vi "real pool auto routine.vi"(0 "ROI Descriptor (Geometric Matching 1)":T4={"Global Rectangle"=[20, 20, 1364, 1012], "Contours"=[{"ID"=enum."External", "Type"=3, "Coordinates"=[20, 20, 1364, 1012]}]} {"Contours"."Type" items=["No Selection", "Point", "Line", "Rectangle", "Oval", "Polygon", "Freehand Region", "Annulus", "Unused2", "Unused3", "Broken Line", "Freehand Line", "Rotated Rectangle"]}, 1 "Settings (Geometric Matching 1)":T3={"Curve Parameters"={"Extraction Mode"=0, "Edge Threshold"=75, "Edge Filter Size"=1, "Min Length"=25, "Row Search Step Size"=15, "Col Search Step Size"=15, "Max Endpoint Gap"=10, "Closed"=FALSE, "Subpixel"=FALSE}, "Match Mode"={"Rotation"=TRUE, "Scale"=FALSE, "Occlusion"=TRUE, "Reserved"=FALSE, "Reserved"=FALSE, "Reserved"=FALSE}, "Range Settings"=[{"Match Constraints"=0, "Min"=0.0, "Max"=360.0}, {"Match Constraints"=2, "Min"=0.0, "Max"=25.0}], "Number of Matches"=1, "Minimum Match Score"=800.0, "SubPixel Accuracy"=FALSE, "Adv. Geometric Match Options 2"=[{"Setup Data Item"=21, "Item Value"=0.0}, {"Setup Data Item"=22, "Item Value"=1.0}]} {"Curve Parameters"."Extraction Mode" items=["Normal", "Uniform Regions"]; "Curve Parameters"."Edge Filter Size" items=["Fine", "Normal", "Contour Tracing"]; "Curve Parameters"."Max Endpoint Gap" min=0; "Curve Parameters"."Col Search Step Size" min=1 max=255 step=1; "Curve Parameters"."Row Search Step Size" min=1 max=255 step=1; "Curve Parameters"."Min Length" min=0; "Curve Parameters"."Edge Threshold" min=1 max=350 step=1; "Range Settings"."Max" format="%.2f"; "Range Settings"."Min" format="%.2f"; "Range Settings"."Match Constraints" items=["Rotation Angle (degrees)", "Scale Factor (%)", "Occlusion (%)"]; "Adv. Geometric Match Options 2"."Setup Data Item" items=["Curve Extraction Mode", "Curve Edge Threshold", "Curve Edge Filter Size", "Min Curve Length", "Curve Row Search Step Size", "Curve Col Search Step Size", "Curve Max Endpoint Gap", "Extract Closed Curves", "Enable Subpixel Curve Extraction", "Enable Correlation Score", "Enable Subpixel Accuracy", "Subpixel Iterations", "Subpixel Tolerance", "Initial Match List Length", "Enable Target Template Curve Score", "Min Match Separation Distance", "Min Match Separation Angle", "Min Match Separation Scale", "Max Match Overlap", "Enable Coarse Result", "Enable Calibration Support", "Enable Contrast Reversal", "Search Strategy", "Refinement Match Factor", "Subpixel Match Factor"]}, 2 "Template File Path (Geometric Matching 1)":path=path "C:/Users/GARLAND/Documents/Projects/Robotics I/Robotics I 3390 2012/Final project/Labview/Real Pool navigation/real pool location templete.png", 3 "ROI Descriptor (Geometric Matching 2)":T4={"Global Rectangle"=[20, 20, 1364, 1012], "Contours"=[{"ID"=enum."External", "Type"=3, "Coordinates"=[20, 20, 1364, 1012]}]} {"Contours"."Type" items=["No Selection", "Point", "Line", "Rectangle", "Oval", "Polygon", "Freehand Region", "Annulus", "Unused2", "Unused3", "Broken Line", "Freehand Line", "Rotated Rectangle"]}, 4 "Settings (Geometric Matching 2)":T3={"Curve Parameters"={"Extraction Mode"=0, "Edge Threshold"=75, "Edge Filter Size"=1, "Min Length"=25, "Row Search Step Size"=15, "Col Search Step Size"=15, "Max Endpoint Gap"=10, "Closed"=FALSE, "Subpixel"=FALSE}, "Match Mode"={"Rotation"=TRUE, "Scale"=FALSE, "Occlusion"=TRUE, "Reserved"=FALSE, "Reserved"=FALSE, "Reserved"=FALSE}, "Range Settings"=[{"Match Constraints"=0, "Min"=0.0, "Max"=360.0}, {"Match Constraints"=2, "Min"=0.0, "Max"=25.0}], "Number of Matches"=1, "Minimum Match Score"=800.0, "SubPixel Accuracy"=FALSE, "Adv. Geometric Match Options 2"=[{"Setup Data Item"=21, "Item Value"=0.0}, {"Setup Data Item"=22, "Item Value"=1.0}]} {"Curve Parameters"."Extraction Mode" items=["Normal", "Uniform Regions"]; "Curve Parameters"."Edge Filter Size" items=["Fine", "Normal", "Contour Tracing"]; "Curve Parameters"."Max Endpoint Gap" min=0; "Curve Parameters"."Col Search Step Size" min=1 max=255 step=1; "Curve Parameters"."Row Search Step Size" min=1 max=255 step=1; "Curve Parameters"."Min Length" min=0; "Curve Parameters"."Edge Threshold" min=1 max=350 step=1; "Range Settings"."Max" format="%.2f"; "Range Settings"."Min" format="%.2f"; "Range Settings"."Match Constraints" items=["Rotation Angle (degrees)", "Scale Factor (%)", "Occlusion (%)"]; "Adv. Geometric Match Options 2"."Setup Data Item" items=["Curve Extraction Mode", "Curve Edge Threshold", "Curve Edge Filter Size", "Min Curve Length", "Curve Row Search Step Size", "Curve Col Search Step Size", "Curve Max Endpoint Gap", "Extract Closed Curves", "Enable Subpixel Curve Extraction", "Enable Correlation Score", "Enable Subpixel Accuracy", "Subpixel Iterations", "Subpixel Tolerance", "Initial Match List Length", "Enable Target Template Curve Score", "Min Match Separation Distance", "Min Match Separation Angle", "Min Match Separation Scale", "Max Match Overlap", "Enable Coarse Result", "Enable Calibration Support", "Enable Contrast Reversal", "Search Strategy", "Refinement Match Factor", "Subpixel Match Factor"]}, 5 "Template File Path (Geometric Matching 2)":path=path "C:/Users/GARLAND/Documents/Projects/Robotics I/Robotics I 3390 2012/Final project/Labview/Real Pool navigation/real pool boat templete.png", 6 "ROI Descriptor (Geometric Matching 3)":T4={"Global Rectangle"=[20, 20, 1364, 1012], "Contours"=[{"ID"=enum."External", "Type"=3, "Coordinates"=[20, 20, 1364, 1012]}]} {"Contours"."Type" items=["No Selection", "Point", "Line", "Rectangle", "Oval", "Polygon", "Freehand Region", "Annulus", "Unused2", "Unused3", "Broken Line", "Freehand Line", "Rotated Rectangle"]}, 7 "error in":errorcluster, 8 "Settings (Geometric Matching 3)":T3={"Curve Parameters"={"Extraction Mode"=0, "Edge Threshold"=75, "Edge Filter Size"=1, "Min Length"=25, "Row Search Step Size"=15, "Col Search Step Size"=15, "Max Endpoint Gap"=10, "Closed"=FALSE, "Subpixel"=FALSE}, "Match Mode"={"Rotation"=TRUE, "Scale"=FALSE, "Occlusion"=TRUE, "Reserved"=FALSE, "Reserved"=FALSE, "Reserved"=FALSE}, "Range Settings"=[{"Match Constraints"=0, "Min"=0.0, "Max"=360.0}, {"Match Constraints"=2, "Min"=0.0, "Max"=25.0}], "Number of Matches"=1, "Minimum Match Score"=800.0, "SubPixel Accuracy"=FALSE, "Adv. Geometric Match Options 2"=[{"Setup Data Item"=21, "Item Value"=0.0}, {"Setup Data Item"=22, "Item Value"=1.0}]} {"Curve Parameters"."Extraction Mode" items=["Normal", "Uniform Regions"]; "Curve Parameters"."Edge Filter Size" items=["Fine", "Normal", "Contour Tracing"]; "Curve Parameters"."Max Endpoint Gap" min=0; "Curve Parameters"."Col Search Step Size" min=1 max=255 step=1; "Curve Parameters"."Row Search Step Size" min=1 max=255 step=1; "Curve Parameters"."Min Length" min=0; "Curve Parameters"."Edge Threshold" min=1 max=350 step=1; "Range Settings"."Max" format="%.2f"; "Range Settings"."Min" format="%.2f"; "Range Settings"."Match Constraints" items=["Rotation Angle (degrees)", "Scale Factor (%)", "Occlusion (%)"]; "Adv. Geometric Match Options 2"."Setup Data Item" items=["Curve Extraction Mode", "Curve Edge Threshold", "Curve Edge Filter Size", "Min Curve Length", "Curve Row Search Step Size", "Curve Col Search Step Size", "Curve Max Endpoint Gap", "Extract Closed Curves", "Enable Subpixel Curve Extraction", "Enable Correlation Score", "Enable Subpixel Accuracy", "Subpixel Iterations", "Subpixel Tolerance", "Initial Match List Length", "Enable Target Template Curve Score", "Min Match Separation Distance", "Min Match Separation Angle", "Min Match Separation Scale", "Max Match Overlap", "Enable Coarse Result", "Enable Calibration Support", "Enable Contrast Reversal", "Search Strategy", "Refinement Match Factor", "Subpixel Match Factor"]}, 9 "Template File Path (Geometric Matching 3)":path=path "C:/Users/GARLAND/Documents/Projects/Robotics I/Robotics I 3390 2012/Final project/Labview/Real Pool navigation/real pool bouy templete.png", 10 "ROI Descriptor (Geometric Matching 4)":T4={"Global Rectangle"=[20, 20, 1364, 1012], "Contours"=[{"ID"=enum."External", "Type"=3, "Coordinates"=[20, 20, 1364, 1012]}]} {"Contours"."Type" items=["No Selection", "Point", "Line", "Rectangle", "Oval", "Polygon", "Freehand Region", "Annulus", "Unused2", "Unused3", "Broken Line", "Freehand Line", "Rotated Rectangle"]}, 11 "Settings (Geometric Matching 4)":T3={"Curve Parameters"={"Extraction Mode"=0, "Edge Threshold"=75, "Edge Filter Size"=1, "Min Length"=25, "Row Search Step Size"=15, "Col Search Step Size"=15, "Max Endpoint Gap"=10, "Closed"=FALSE, "Subpixel"=FALSE}, "Match Mode"={"Rotation"=TRUE, "Scale"=FALSE, "Occlusion"=TRUE, "Reserved"=FALSE, "Reserved"=FALSE, "Reserved"=FALSE}, "Range Settings"=[{"Match Constraints"=0, "Min"=0.0, "Max"=360.0}, {"Match Constraints"=2, "Min"=0.0, "Max"=25.0}], "Number of Matches"=1, "Minimum Match Score"=800.0, "SubPixel Accuracy"=FALSE, "Adv. Geometric Match Options 2"=[{"Setup Data Item"=21, "Item Value"=0.0}, {"Setup Data Item"=22, "Item Value"=1.0}]} {"Curve Parameters"."Extraction Mode" items=["Normal", "Uniform Regions"]; "Curve Parameters"."Edge Filter Size" items=["Fine", "Normal", "Contour Tracing"]; "Curve Parameters"."Max Endpoint Gap" min=0; "Curve Parameters"."Col Search Step Size" min=1 max=255 step=1; "Curve Parameters"."Row Search Step Size" min=1 max=255 step=1; "Curve Parameters"."Min Length" min=0; "Curve Parameters"."Edge Threshold" min=1 max=350 step=1; "Range Settings"."Max" format="%.2f"; "Range Settings"."Min" format="%.2f"; "Range Settings"."Match Constraints" items=["Rotation Angle (degrees)", "Scale Factor (%)", "Occlusion (%)"]; "Adv. Geometric Match Options 2"."Setup Data Item" items=["Curve Extraction Mode", "Curve Edge Threshold", "Curve Edge Filter Size", "Min Curve Length", "Curve Row Search Step Size", "Curve Col Search Step Size", "Curve Max Endpoint Gap", "Extract Closed Curves", "Enable Subpixel Curve Extraction", "Enable Correlation Score", "Enable Subpixel Accuracy", "Subpixel Iterations", "Subpixel Tolerance", "Initial Match List Length", "Enable Target Template Curve Score", "Min Match Separation Distance", "Min Match Separation Angle", "Min Match Separation Scale", "Max Match Overlap", "Enable Coarse Result", "Enable Calibration Support", "Enable Contrast Reversal", "Search Strategy", "Refinement Match Factor", "Subpixel Match Factor"]}, 12 "Template File Path (Geometric Matching 4)":path=path "C:/Users/GARLAND/Documents/Projects/Robotics I/Robotics I 3390 2012/Final project/Labview/Real Pool navigation/real pool whale templete.png", 13 "ROI Descriptor (Geometric Matching 5)":T4={"Global Rectangle"=[20, 20, 1364, 1012], "Contours"=[{"ID"=enum."External", "Type"=3, "Coordinates"=[20, 20, 1364, 1012]}]} {"Contours"."Type" items=["No Selection", "Point", "Line", "Rectangle", "Oval", "Polygon", "Freehand Region", "Annulus", "Unused2", "Unused3", "Broken Line", "Freehand Line", "Rotated Rectangle"]}, 14 "Settings (Geometric Matching 5)":T3={"Curve Parameters"={"Extraction Mode"=0, "Edge Threshold"=75, "Edge Filter Size"=1, "Min Length"=25, "Row Search Step Size"=15, "Col Search Step Size"=15, "Max Endpoint Gap"=10, "Closed"=FALSE, "Subpixel"=FALSE}, "Match Mode"={"Rotation"=TRUE, "Scale"=FALSE, "Occlusion"=TRUE, "Reserved"=FALSE, "Reserved"=FALSE, "Reserved"=FALSE}, "Range Settings"=[{"Match Constraints"=0, "Min"=0.0, "Max"=360.0}, {"Match Constraints"=2, "Min"=0.0, "Max"=25.0}], "Number of Matches"=1, "Minimum Match Score"=800.0, "SubPixel Accuracy"=FALSE, "Adv. Geometric Match Options 2"=[{"Setup Data Item"=21, "Item Value"=0.0}, {"Setup Data Item"=22, "Item Value"=1.0}]} {"Curve Parameters"."Extraction Mode" items=["Normal", "Uniform Regions"]; "Curve Parameters"."Edge Filter Size" items=["Fine", "Normal", "Contour Tracing"]; "Curve Parameters"."Max Endpoint Gap" min=0; "Curve Parameters"."Col Search Step Size" min=1 max=255 step=1; "Curve Parameters"."Row Search Step Size" min=1 max=255 step=1; "Curve Parameters"."Min Length" min=0; "Curve Parameters"."Edge Threshold" min=1 max=350 step=1; "Range Settings"."Max" format="%.2f"; "Range Settings"."Min" format="%.2f"; "Range Settings"."Match Constraints" items=["Rotation Angle (degrees)", "Scale Factor (%)", "Occlusion (%)"]; "Adv. Geometric Match Options 2"."Setup Data Item" items=["Curve Extraction Mode", "Curve Edge Threshold", "Curve Edge Filter Size", "Min Curve Length", "Curve Row Search Step Size", "Curve Col Search Step Size", "Curve Max Endpoint Gap", "Extract Closed Curves", "Enable Subpixel Curve Extraction", "Enable Correlation Score", "Enable Subpixel Accuracy", "Subpixel Iterations", "Subpixel Tolerance", "Initial Match List Length", "Enable Target Template Curve Score", "Min Match Separation Distance", "Min Match Separation Angle", "Min Match Separation Scale", "Max Match Overlap", "Enable Coarse Result", "Enable Calibration Support", "Enable Contrast Reversal", "Search Strategy", "Refinement Match Factor", "Subpixel Match Factor"]}, 15 "Template File Path (Geometric Matching 5)":path=path "C:/Users/GARLAND/Documents/Projects/Robotics I/Robotics I 3390 2012/Final project/Labview/Real Pool navigation/real pool square templete.png", 16 "ROI Descriptor (Geometric Matching 6)":T4={"Global Rectangle"=[20, 20, 1364, 1012], "Contours"=[{"ID"=enum."External", "Type"=3, "Coordinates"=[20, 20, 1364, 1012]}]} {"Contours"."Type" items=["No Selection", "Point", "Line", "Rectangle", "Oval", "Polygon", "Freehand Region", "Annulus", "Unused2", "Unused3", "Broken Line", "Freehand Line", "Rotated Rectangle"]}, 17 "Settings (Geometric Matching 6)":T3={"Curve Parameters"={"Extraction Mode"=0, "Edge Threshold"=75, "Edge Filter Size"=1, "Min Length"=25, "Row Search Step Size"=15, "Col Search Step Size"=15, "Max Endpoint Gap"=10, "Closed"=FALSE, "Subpixel"=FALSE}, "Match Mode"={"Rotation"=TRUE, "Scale"=FALSE, "Occlusion"=TRUE, "Reserved"=FALSE, "Reserved"=FALSE, "Reserved"=FALSE}, "Range Settings"=[{"Match Constraints"=0, "Min"=0.0, "Max"=360.0}, {"Match Constraints"=2, "Min"=0.0, "Max"=25.0}], "Number of Matches"=1, "Minimum Match Score"=800.0, "SubPixel Accuracy"=FALSE, "Adv. Geometric Match Options 2"=[{"Setup Data Item"=21, "Item Value"=0.0}, {"Setup Data Item"=22, "Item Value"=1.0}]} {"Curve Parameters"."Extraction Mode" items=["Normal", "Uniform Regions"]; "Curve Parameters"."Edge Filter Size" items=["Fine", "Normal", "Contour Tracing"]; "Curve Parameters"."Max Endpoint Gap" min=0; "Curve Parameters"."Col Search Step Size" min=1 max=255 step=1; "Curve Parameters"."Row Search Step Size" min=1 max=255 step=1; "Curve Parameters"."Min Length" min=0; "Curve Parameters"."Edge Threshold" min=1 max=350 step=1; "Range Settings"."Max" format="%.2f"; "Range Settings"."Min" format="%.2f"; "Range Settings"."Match Constraints" items=["Rotation Angle (degrees)", "Scale Factor (%)", "Occlusion (%)"]; "Adv. Geometric Match Options 2"."Setup Data Item" items=["Curve Extraction Mode", "Curve Edge Threshold", "Curve Edge Filter Size", "Min Curve Length", "Curve Row Search Step Size", "Curve Col Search Step Size", "Curve Max Endpoint Gap", "Extract Closed Curves", "Enable Subpixel Curve Extraction", "Enable Correlation Score", "Enable Subpixel Accuracy", "Subpixel Iterations", "Subpixel Tolerance", "Initial Match List Length", "Enable Target Template Curve Score", "Min Match Separation Distance", "Min Match Separation Angle", "Min Match Separation Scale", "Max Match Overlap", "Enable Coarse Result", "Enable Calibration Support", "Enable Contrast Reversal", "Search Strategy", "Refinement Match Factor", "Subpixel Match Factor"]}, 18 "Template File Path (Geometric Matching 6)":path=path "C:/Users/GARLAND/Documents/Projects/Robotics I/Robotics I 3390 2012/Final project/Labview/Real Pool navigation/real pool big boat templete.png") -> (20 "Matches (Geometric Matching 1)":T6[](array[typedef]) {"Correlation Score" format="%.2f"; "Target Template Curve Score" format="%.2f"; "Template Target Curve Score" format="%.2f"; "Bounding Box"."y" format="%.2f"; "Bounding Box"."x" format="%.2f"; "Position"."y" format="%.2f"; "Position"."x" format="%.2f"; "Score" format="%.2f"; "Scale" format="%.2f"; "Angle" format="%.2f"; "Occlusion %" format="%.2f"}, 21 "Matches (Geometric Matching 2)":T6[](array[typedef]) {"Correlation Score" format="%.2f"; "Target Template Curve Score" format="%.2f"; "Template Target Curve Score" format="%.2f"; "Bounding Box"."y" format="%.2f"; "Bounding Box"."x" format="%.2f"; "Position"."y" format="%.2f"; "Position"."x" format="%.2f"; "Score" format="%.2f"; "Scale" format="%.2f"; "Angle" format="%.2f"; "Occlusion %" format="%.2f"}, 22 "Matches (Geometric Matching 3)":T6[](array[typedef]) {"Correlation Score" format="%.2f"; "Target Template Curve Score" format="%.2f"; "Template Target Curve Score" format="%.2f"; "Bounding Box"."y" format="%.2f"; "Bounding Box"."x" format="%.2f"; "Position"."y" format="%.2f"; "Position"."x" format="%.2f"; "Score" format="%.2f"; "Scale" format="%.2f"; "Angle" format="%.2f"; "Occlusion %" format="%.2f"}, 23 "Matches (Geometric Matching 4)":T6[](array[typedef]) {"Correlation Score" format="%.2f"; "Target Template Curve Score" format="%.2f"; "Template Target Curve Score" format="%.2f"; "Bounding Box"."y" format="%.2f"; "Bounding Box"."x" format="%.2f"; "Position"."y" format="%.2f"; "Position"."x" format="%.2f"; "Score" format="%.2f"; "Scale" format="%.2f"; "Angle" format="%.2f"; "Occlusion %" format="%.2f"}, 24 "Matches (Geometric Matching 5)":T6[](array[typedef]) {"Correlation Score" format="%.2f"; "Target Template Curve Score" format="%.2f"; "Template Target Curve Score" format="%.2f"; "Bounding Box"."y" format="%.2f"; "Bounding Box"."x" format="%.2f"; "Position"."y" format="%.2f"; "Position"."x" format="%.2f"; "Score" format="%.2f"; "Scale" format="%.2f"; "Angle" format="%.2f"; "Occlusion %" format="%.2f"}, 25 "Matches (Geometric Matching 6)":T6[](array[typedef]) {"Correlation Score" format="%.2f"; "Target Template Curve Score" format="%.2f"; "Template Target Curve Score" format="%.2f"; "Bounding Box"."y" format="%.2f"; "Bounding Box"."x" format="%.2f"; "Position"."y" format="%.2f"; "Position"."x" format="%.2f"; "Score" format="%.2f"; "Scale" format="%.2f"; "Angle" format="%.2f"; "Occlusion %" format="%.2f"}, 27 "error out":errorcluster)   [LabVIEW 2011]
uses:
  <vilib>/vision/Pattern Matching.llb/IMAQ GM Match Report.ctl
  <vilib>/vision/Pattern Matching.llb/IMAQ Curve Parameters.ctl
  <vilib>/vision/Pattern Matching.llb/IMAQ Match Range Setting.ctl
panel:
  out "Image Out":T5(plugin-control)
  # "Range"
  # "Range"
  # "Range"
  # "Range"
  # "Range"
  # "Range"
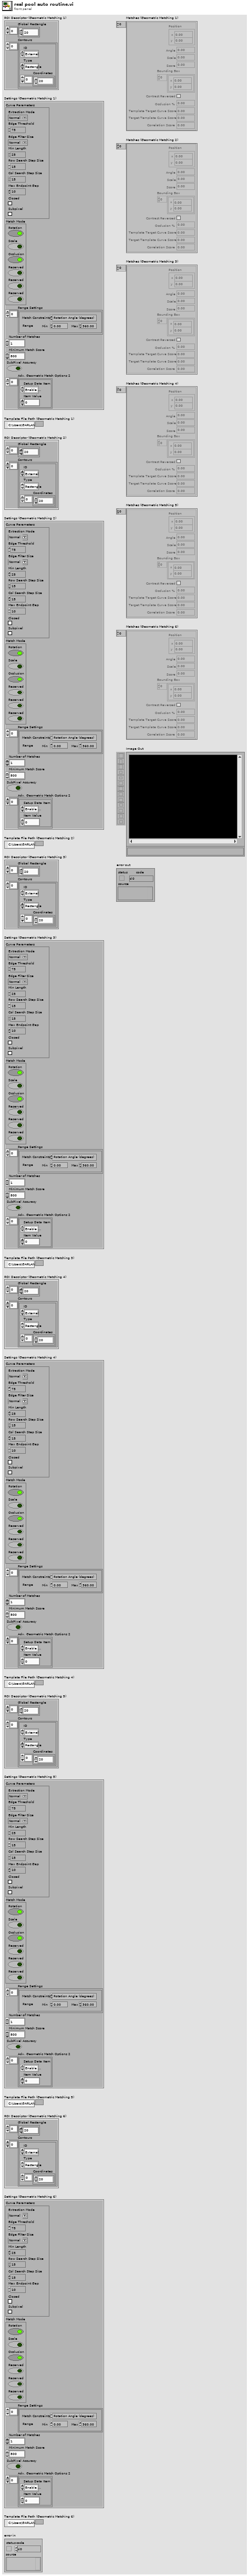
[diagram p1: front panel]
types:
  T1 = typedef "IMAQ Curve Parameters.ctl" = cluster{"Extraction Mode":u32, "Edge Threshold":i32, "Edge Filter Size":u32, "Min Length":i32, "Row Search Step Size":i32, "Col Search Step Size":i32, "Max Endpoint Gap":i32, "Closed":bool, "Subpixel":bool}
  T2 = typedef "IMAQ Match Range Setting.ctl" = cluster{"Match Constraints":u32, "Min":dbl, "Max":dbl}
  T3 = cluster{"Curve Parameters":T1, "Match Mode":cluster{"Rotation":bool, "Scale":bool, "Occlusion":bool, "Reserved":bool, "Reserved":bool, "Reserved":bool}, "Range Settings":T2[], "Number of Matches":i32, "Minimum Match Score":sgl, "SubPixel Accuracy":bool, "Adv. Geometric Match Options 2":cluster{"Setup Data Item":u16, "Item Value":dbl}[]}
  T4 = cluster{"Global Rectangle":i32[], "Contours":cluster{"ID":enum32{"External", "Internal"}, "Type":u32, "Coordinates":i32[]}[]}
  T5 = typedef "IMAQ Image.ctl" = refnum<image>
  T6 = typedef "IMAQ GM Match Report.ctl" = cluster{"Position":cluster{"x":sgl, "y":sgl}, "Angle":sgl, "Scale":sgl, "Score":sgl, "Bounding Box":cluster{"x":sgl, "y":sgl}[], "Contrast Reversed":bool, "Occlusion %":sgl, "Template Target Curve Score":sgl, "Target Template Curve Score":sgl, "Correlation Score":sgl}
  T7 = typedef "Image Type" = u32
diagram:
  w2 = u32 0 items=["Grayscale", "Binary", "Gradient", "Rainbow", "Temperature", "User Defined"] ("Palette")
  w4 = "Geometric Matching 6" ("Step Name")
  w15 = "Geometric Matching 5" ("Step Name")
  w26 = "Geometric Matching 4" ("Step Name")
  w37 = "Geometric Matching 3" ("Step Name")
  w48 = "Geometric Matching 2" ("Step Name")
  w59 = "Geometric Matching 1" ("Step Name")
  w70 = T7 0 items=["Grayscale (U8)", "Grayscale (I16)", "Grayscale (SGL)", "Complex (CSG)", "RGB (U32)", "HSL (U32)", "RGB (U64)", "Grayscale (U16)"] ("Image Type")
  # "Geometric Matching"
  # "Geometric Matching"
  # "Geometric Matching"
  # "Geometric Matching"
  # "Geometric Matching"
  # "Geometric Matching"
  n1 = Call Chain() -> (call chain=w74:string[])
  n2 = Index Array(array=w74) -> (element=w73:string)  [unwired: 1 in]
  n3 = call "File Dialog"("prompt"="Select an image file...") -> ("selected path"=w71:path)  [unwired: 6 in, 8 out]
  n4 = call "IMAQ Create"("Image Name"=w73, "Image Type"=w70, "error in (no error)"="error in") -> ("New Image"=w77:T5, "error out"=w76:errorcluster)  [unwired: 1 in, 1 out]
  n5 = call "IMAQ ReadFile"("File Path"=w71, "error in (no error)"=w76, "Image"=w77) -> ("error out"=w78:errorcluster, "Image Out"=w67:T5)  [unwired: 2 in, 5 out]
  n6 = Unbundle By Name(w78) -> ("code"=w62:i32)
  n7 = case shown="Default" w62 {
    tunnel: "Template File Path (Geometric Matching 1)" -> [_ w81]
    tunnel: w78 -> [_ w82]
    tunnel: "Settings (Geometric Matching 1)" -> [_ w91]
    tunnel: "ROI Descriptor (Geometric Matching 1)" -> [_ w90]
    tunnel: w67 -> [w79 w85]
    tunnel: [_ w89] -> w66
    tunnel: [_ w88] -> w64
    tunnel: [_ w87] -> w63
    tunnel: [_ w86] -> _
    tunnel: [w79 w85] -> w61
    tunnel: w59 -> [_ w80]
    frame -1074396199, -1074396198 {
      # "Discard Coordinate System Error"
    }
    frame Default {
      n8 = while {
        shift-right: [w100] -> w83
        shift-left: _ -> [w99]
        tunnel: [w97] -> w84
        tunnel: w82 -> [w96]
        tunnel: w81 -> [w92]
        tunnel: w80 -> [w95]
        shift-right: [w92] -> _
        shift-left: _ -> [w94]
        stop <- FALSE continue-if-true
        n9 = Not Equal?(x=w94, y=w92) -> (x != y?=w93:bool)
        n10 = case shown="True" w93 {
          tunnel: [w102 w114] -> w100
          tunnel: w99 -> [w102 w106]
          tunnel: [w101 w111] -> w97
          tunnel: w96 -> [w101 w107]
          tunnel: w95 -> [_ w108]
          tunnel: w92 -> [_ w104]
          frame False {
          }
          frame True {
            n11 = Call Chain() -> (call chain=w110:string[])
            n12 = stacked-sequence {
              tunnel: w107 -> [w118]
              tunnel: w106 -> [w117]
              tunnel: [w118] -> w105
              frame #0 {
                n13 = call "IMAQ Dispose"("Image"=w117) -> ()  [unwired: 2 in, 4 out]
              }
            }
            n14 = Index Array(array=w110) -> (element=w109:string)  [unwired: 1 in]
            n15 = Format Into String(format string="GM2 Template %s %s" ("Image Name"), w109, w108) -> (resulting string=w116:string)  [unwired: 2 in, 1 out]
            n16 = call "IMAQ Create"("Image Name"=w116, "error in (no error)"=w105) -> ("New Image"=w113:T5, "error out"=w112:errorcluster)  [unwired: 2 in, 1 out]
            n17 = call <vilib>:"IVA Get Alternate Path.vi"("Path In"=w104) -> ("Path Out"=w103:path)  [unwired: 10 out]
            n18 = call "IMAQ Read Image And Vision Info"("File Path"=w103, "error in (no error)"=w112, "Image"=w113) -> ("error out"=w111:errorcluster, "Image Out"=w114:T5)  [unwired: 1 in, 6 out]
          }
        }
      }
      n19 = call <vilib>:"IVA Match Geometric Pattern Algorithm 3.vi"("Template"=w83, "error in (no error)"=w84, "Settings"=w91, "ROI Descriptor"=w90, "Image"=w85) -> ("error out"=w89:errorcluster, "Calibrated Matches"=w87:T6[], "Matches"=w88:T6[], "Number of Matches"=w86:i32)  [unwired: 3 out]
    }
  }
  "Matches (Geometric Matching 1)" <- w64
  n20 = call <vilib>:"IVA Store Match Geometric Pattern Results.vi"("Calibrated Matches"=w63, "error in (no error)"=w66, "Matches"=w64, "Step Name"=w59, "Image in"=w61) -> ("error out"=w65:errorcluster, "Image dup"=w56:T5)  [unwired: 5 out]
  n21 = Unbundle By Name(w65) -> ("code"=w51:i32)
  n22 = case shown="Default" w51 {
    tunnel: "Template File Path (Geometric Matching 2)" -> [_ w121]
    tunnel: w65 -> [_ w122]
    tunnel: "Settings (Geometric Matching 2)" -> [_ w131]
    tunnel: "ROI Descriptor (Geometric Matching 2)" -> [_ w130]
    tunnel: w56 -> [w119 w125]
    tunnel: [_ w129] -> w55
    tunnel: [_ w128] -> w53
    tunnel: [_ w127] -> w52
    tunnel: [_ w126] -> _
    tunnel: [w119 w125] -> w50
    tunnel: w48 -> [_ w120]
    frame -1074396199, -1074396198 {
      # "Discard Coordinate System Error"
    }
    frame Default {
      n23 = while {
        shift-right: [w140] -> w123
        shift-left: _ -> [w139]
        tunnel: [w137] -> w124
        tunnel: w122 -> [w136]
        tunnel: w121 -> [w132]
        tunnel: w120 -> [w135]
        shift-right: [w132] -> _
        shift-left: _ -> [w134]
        stop <- FALSE continue-if-true
        n24 = Not Equal?(x=w134, y=w132) -> (x != y?=w133:bool)
        n25 = case shown="True" w133 {
          tunnel: [w142 w154] -> w140
          tunnel: w139 -> [w142 w146]
          tunnel: [w141 w151] -> w137
          tunnel: w136 -> [w141 w147]
          tunnel: w135 -> [_ w148]
          tunnel: w132 -> [_ w144]
          frame False {
          }
          frame True {
            n26 = Call Chain() -> (call chain=w150:string[])
            n27 = stacked-sequence {
              tunnel: w147 -> [w158]
              tunnel: w146 -> [w157]
              tunnel: [w158] -> w145
              frame #0 {
                n28 = call "IMAQ Dispose"("Image"=w157) -> ()  [unwired: 2 in, 4 out]
              }
            }
            n29 = Index Array(array=w150) -> (element=w149:string)  [unwired: 1 in]
            n30 = Format Into String(format string="GM2 Template %s %s" ("Image Name"), w149, w148) -> (resulting string=w156:string)  [unwired: 2 in, 1 out]
            n31 = call "IMAQ Create"("Image Name"=w156, "error in (no error)"=w145) -> ("New Image"=w153:T5, "error out"=w152:errorcluster)  [unwired: 2 in, 1 out]
            n32 = call <vilib>:"IVA Get Alternate Path.vi"("Path In"=w144) -> ("Path Out"=w143:path)  [unwired: 10 out]
            n33 = call "IMAQ Read Image And Vision Info"("File Path"=w143, "error in (no error)"=w152, "Image"=w153) -> ("error out"=w151:errorcluster, "Image Out"=w154:T5)  [unwired: 1 in, 6 out]
          }
        }
      }
      n34 = call <vilib>:"IVA Match Geometric Pattern Algorithm 3.vi"("Template"=w123, "error in (no error)"=w124, "Settings"=w131, "ROI Descriptor"=w130, "Image"=w125) -> ("error out"=w129:errorcluster, "Calibrated Matches"=w127:T6[], "Matches"=w128:T6[], "Number of Matches"=w126:i32)  [unwired: 3 out]
    }
  }
  "Matches (Geometric Matching 2)" <- w53
  n35 = call <vilib>:"IVA Store Match Geometric Pattern Results.vi"("Calibrated Matches"=w52, "error in (no error)"=w55, "Matches"=w53, "Step Name"=w48, "Image in"=w50) -> ("error out"=w54:errorcluster, "Image dup"=w45:T5)  [unwired: 5 out]
  n36 = Unbundle By Name(w54) -> ("code"=w40:i32)
  n37 = case shown="Default" w40 {
    tunnel: "Template File Path (Geometric Matching 3)" -> [_ w161]
    tunnel: w54 -> [_ w162]
    tunnel: "Settings (Geometric Matching 3)" -> [_ w171]
    tunnel: "ROI Descriptor (Geometric Matching 3)" -> [_ w170]
    tunnel: w45 -> [w159 w165]
    tunnel: [_ w169] -> w44
    tunnel: [_ w168] -> w42
    tunnel: [_ w167] -> w41
    tunnel: [_ w166] -> _
    tunnel: [w159 w165] -> w39
    tunnel: w37 -> [_ w160]
    frame -1074396199, -1074396198 {
      # "Discard Coordinate System Error"
    }
    frame Default {
      n38 = while {
        shift-right: [w180] -> w163
        shift-left: _ -> [w179]
        tunnel: [w177] -> w164
        tunnel: w162 -> [w176]
        tunnel: w161 -> [w172]
        tunnel: w160 -> [w175]
        shift-right: [w172] -> _
        shift-left: _ -> [w174]
        stop <- FALSE continue-if-true
        n39 = Not Equal?(x=w174, y=w172) -> (x != y?=w173:bool)
        n40 = case shown="True" w173 {
          tunnel: [w182 w194] -> w180
          tunnel: w179 -> [w182 w186]
          tunnel: [w181 w191] -> w177
          tunnel: w176 -> [w181 w187]
          tunnel: w175 -> [_ w188]
          tunnel: w172 -> [_ w184]
          frame False {
          }
          frame True {
            n41 = Call Chain() -> (call chain=w190:string[])
            n42 = stacked-sequence {
              tunnel: w187 -> [w198]
              tunnel: w186 -> [w197]
              tunnel: [w198] -> w185
              frame #0 {
                n43 = call "IMAQ Dispose"("Image"=w197) -> ()  [unwired: 2 in, 4 out]
              }
            }
            n44 = Index Array(array=w190) -> (element=w189:string)  [unwired: 1 in]
            n45 = Format Into String(format string="GM2 Template %s %s" ("Image Name"), w189, w188) -> (resulting string=w196:string)  [unwired: 2 in, 1 out]
            n46 = call "IMAQ Create"("Image Name"=w196, "error in (no error)"=w185) -> ("New Image"=w193:T5, "error out"=w192:errorcluster)  [unwired: 2 in, 1 out]
            n47 = call <vilib>:"IVA Get Alternate Path.vi"("Path In"=w184) -> ("Path Out"=w183:path)  [unwired: 10 out]
            n48 = call "IMAQ Read Image And Vision Info"("File Path"=w183, "error in (no error)"=w192, "Image"=w193) -> ("error out"=w191:errorcluster, "Image Out"=w194:T5)  [unwired: 1 in, 6 out]
          }
        }
      }
      n49 = call <vilib>:"IVA Match Geometric Pattern Algorithm 3.vi"("Template"=w163, "error in (no error)"=w164, "Settings"=w171, "ROI Descriptor"=w170, "Image"=w165) -> ("error out"=w169:errorcluster, "Calibrated Matches"=w167:T6[], "Matches"=w168:T6[], "Number of Matches"=w166:i32)  [unwired: 3 out]
    }
  }
  "Matches (Geometric Matching 3)" <- w42
  n50 = call <vilib>:"IVA Store Match Geometric Pattern Results.vi"("Calibrated Matches"=w41, "error in (no error)"=w44, "Matches"=w42, "Step Name"=w37, "Image in"=w39) -> ("error out"=w43:errorcluster, "Image dup"=w34:T5)  [unwired: 5 out]
  n51 = Unbundle By Name(w43) -> ("code"=w29:i32)
  n52 = case shown="Default" w29 {
    tunnel: "Template File Path (Geometric Matching 4)" -> [_ w201]
    tunnel: w43 -> [_ w202]
    tunnel: "Settings (Geometric Matching 4)" -> [_ w211]
    tunnel: "ROI Descriptor (Geometric Matching 4)" -> [_ w210]
    tunnel: w34 -> [w199 w205]
    tunnel: [_ w209] -> w33
    tunnel: [_ w208] -> w31
    tunnel: [_ w207] -> w30
    tunnel: [_ w206] -> _
    tunnel: [w199 w205] -> w28
    tunnel: w26 -> [_ w200]
    frame -1074396199, -1074396198 {
      # "Discard Coordinate System Error"
    }
    frame Default {
      n53 = while {
        shift-right: [w220] -> w203
        shift-left: _ -> [w219]
        tunnel: [w217] -> w204
        tunnel: w202 -> [w216]
        tunnel: w201 -> [w212]
        tunnel: w200 -> [w215]
        shift-right: [w212] -> _
        shift-left: _ -> [w214]
        stop <- FALSE continue-if-true
        n54 = Not Equal?(x=w214, y=w212) -> (x != y?=w213:bool)
        n55 = case shown="True" w213 {
          tunnel: [w222 w234] -> w220
          tunnel: w219 -> [w222 w226]
          tunnel: [w221 w231] -> w217
          tunnel: w216 -> [w221 w227]
          tunnel: w215 -> [_ w228]
          tunnel: w212 -> [_ w224]
          frame False {
          }
          frame True {
            n56 = Call Chain() -> (call chain=w230:string[])
            n57 = stacked-sequence {
              tunnel: w227 -> [w238]
              tunnel: w226 -> [w237]
              tunnel: [w238] -> w225
              frame #0 {
                n58 = call "IMAQ Dispose"("Image"=w237) -> ()  [unwired: 2 in, 4 out]
              }
            }
            n59 = Index Array(array=w230) -> (element=w229:string)  [unwired: 1 in]
            n60 = Format Into String(format string="GM2 Template %s %s" ("Image Name"), w229, w228) -> (resulting string=w236:string)  [unwired: 2 in, 1 out]
            n61 = call "IMAQ Create"("Image Name"=w236, "error in (no error)"=w225) -> ("New Image"=w233:T5, "error out"=w232:errorcluster)  [unwired: 2 in, 1 out]
            n62 = call <vilib>:"IVA Get Alternate Path.vi"("Path In"=w224) -> ("Path Out"=w223:path)  [unwired: 10 out]
            n63 = call "IMAQ Read Image And Vision Info"("File Path"=w223, "error in (no error)"=w232, "Image"=w233) -> ("error out"=w231:errorcluster, "Image Out"=w234:T5)  [unwired: 1 in, 6 out]
          }
        }
      }
      n64 = call <vilib>:"IVA Match Geometric Pattern Algorithm 3.vi"("Template"=w203, "error in (no error)"=w204, "Settings"=w211, "ROI Descriptor"=w210, "Image"=w205) -> ("error out"=w209:errorcluster, "Calibrated Matches"=w207:T6[], "Matches"=w208:T6[], "Number of Matches"=w206:i32)  [unwired: 3 out]
    }
  }
  "Matches (Geometric Matching 4)" <- w31
  n65 = call <vilib>:"IVA Store Match Geometric Pattern Results.vi"("Calibrated Matches"=w30, "error in (no error)"=w33, "Matches"=w31, "Step Name"=w26, "Image in"=w28) -> ("error out"=w32:errorcluster, "Image dup"=w23:T5)  [unwired: 5 out]
  n66 = Unbundle By Name(w32) -> ("code"=w18:i32)
  n67 = case shown="Default" w18 {
    tunnel: "Template File Path (Geometric Matching 5)" -> [_ w241]
    tunnel: w32 -> [_ w242]
    tunnel: "Settings (Geometric Matching 5)" -> [_ w251]
    tunnel: "ROI Descriptor (Geometric Matching 5)" -> [_ w250]
    tunnel: w23 -> [w239 w245]
    tunnel: [_ w249] -> w22
    tunnel: [_ w248] -> w20
    tunnel: [_ w247] -> w19
    tunnel: [_ w246] -> _
    tunnel: [w239 w245] -> w17
    tunnel: w15 -> [_ w240]
    frame -1074396199, -1074396198 {
      # "Discard Coordinate System Error"
    }
    frame Default {
      n68 = while {
        shift-right: [w260] -> w243
        shift-left: _ -> [w259]
        tunnel: [w257] -> w244
        tunnel: w242 -> [w256]
        tunnel: w241 -> [w252]
        tunnel: w240 -> [w255]
        shift-right: [w252] -> _
        shift-left: _ -> [w254]
        stop <- FALSE continue-if-true
        n69 = Not Equal?(x=w254, y=w252) -> (x != y?=w253:bool)
        n70 = case shown="True" w253 {
          tunnel: [w262 w274] -> w260
          tunnel: w259 -> [w262 w266]
          tunnel: [w261 w271] -> w257
          tunnel: w256 -> [w261 w267]
          tunnel: w255 -> [_ w268]
          tunnel: w252 -> [_ w264]
          frame False {
          }
          frame True {
            n71 = Call Chain() -> (call chain=w270:string[])
            n72 = stacked-sequence {
              tunnel: w267 -> [w278]
              tunnel: w266 -> [w277]
              tunnel: [w278] -> w265
              frame #0 {
                n73 = call "IMAQ Dispose"("Image"=w277) -> ()  [unwired: 2 in, 4 out]
              }
            }
            n74 = Index Array(array=w270) -> (element=w269:string)  [unwired: 1 in]
            n75 = Format Into String(format string="GM2 Template %s %s" ("Image Name"), w269, w268) -> (resulting string=w276:string)  [unwired: 2 in, 1 out]
            n76 = call "IMAQ Create"("Image Name"=w276, "error in (no error)"=w265) -> ("New Image"=w273:T5, "error out"=w272:errorcluster)  [unwired: 2 in, 1 out]
            n77 = call <vilib>:"IVA Get Alternate Path.vi"("Path In"=w264) -> ("Path Out"=w263:path)  [unwired: 10 out]
            n78 = call "IMAQ Read Image And Vision Info"("File Path"=w263, "error in (no error)"=w272, "Image"=w273) -> ("error out"=w271:errorcluster, "Image Out"=w274:T5)  [unwired: 1 in, 6 out]
          }
        }
      }
      n79 = call <vilib>:"IVA Match Geometric Pattern Algorithm 3.vi"("Template"=w243, "error in (no error)"=w244, "Settings"=w251, "ROI Descriptor"=w250, "Image"=w245) -> ("error out"=w249:errorcluster, "Calibrated Matches"=w247:T6[], "Matches"=w248:T6[], "Number of Matches"=w246:i32)  [unwired: 3 out]
    }
  }
  "Matches (Geometric Matching 5)" <- w20
  n80 = call <vilib>:"IVA Store Match Geometric Pattern Results.vi"("Calibrated Matches"=w19, "error in (no error)"=w22, "Matches"=w20, "Step Name"=w15, "Image in"=w17) -> ("error out"=w21:errorcluster, "Image dup"=w12:T5)  [unwired: 5 out]
  n81 = Unbundle By Name(w21) -> ("code"=w7:i32)
  n82 = case shown="Default" w7 {
    tunnel: "Template File Path (Geometric Matching 6)" -> [_ w281]
    tunnel: w21 -> [_ w282]
    tunnel: "Settings (Geometric Matching 6)" -> [_ w291]
    tunnel: "ROI Descriptor (Geometric Matching 6)" -> [_ w290]
    tunnel: w12 -> [w279 w285]
    tunnel: [_ w289] -> w11
    tunnel: [_ w288] -> w9
    tunnel: [_ w287] -> w8
    tunnel: [_ w286] -> _
    tunnel: [w279 w285] -> w6
    tunnel: w4 -> [_ w280]
    frame -1074396199, -1074396198 {
      # "Discard Coordinate System Error"
    }
    frame Default {
      n83 = while {
        shift-right: [w300] -> w283
        shift-left: _ -> [w299]
        tunnel: [w297] -> w284
        tunnel: w282 -> [w296]
        tunnel: w281 -> [w292]
        tunnel: w280 -> [w295]
        shift-right: [w292] -> _
        shift-left: _ -> [w294]
        stop <- FALSE continue-if-true
        n84 = Not Equal?(x=w294, y=w292) -> (x != y?=w293:bool)
        n85 = case shown="True" w293 {
          tunnel: [w302 w314] -> w300
          tunnel: w299 -> [w302 w306]
          tunnel: [w301 w311] -> w297
          tunnel: w296 -> [w301 w307]
          tunnel: w295 -> [_ w308]
          tunnel: w292 -> [_ w304]
          frame False {
          }
          frame True {
            n86 = Call Chain() -> (call chain=w310:string[])
            n87 = stacked-sequence {
              tunnel: w307 -> [w318]
              tunnel: w306 -> [w317]
              tunnel: [w318] -> w305
              frame #0 {
                n88 = call "IMAQ Dispose"("Image"=w317) -> ()  [unwired: 2 in, 4 out]
              }
            }
            n89 = Index Array(array=w310) -> (element=w309:string)  [unwired: 1 in]
            n90 = Format Into String(format string="GM2 Template %s %s" ("Image Name"), w309, w308) -> (resulting string=w316:string)  [unwired: 2 in, 1 out]
            n91 = call "IMAQ Create"("Image Name"=w316, "error in (no error)"=w305) -> ("New Image"=w313:T5, "error out"=w312:errorcluster)  [unwired: 2 in, 1 out]
            n92 = call <vilib>:"IVA Get Alternate Path.vi"("Path In"=w304) -> ("Path Out"=w303:path)  [unwired: 10 out]
            n93 = call "IMAQ Read Image And Vision Info"("File Path"=w303, "error in (no error)"=w312, "Image"=w313) -> ("error out"=w311:errorcluster, "Image Out"=w314:T5)  [unwired: 1 in, 6 out]
          }
        }
      }
      n94 = call <vilib>:"IVA Match Geometric Pattern Algorithm 3.vi"("Template"=w283, "error in (no error)"=w284, "Settings"=w291, "ROI Descriptor"=w290, "Image"=w285) -> ("error out"=w289:errorcluster, "Calibrated Matches"=w287:T6[], "Matches"=w288:T6[], "Number of Matches"=w286:i32)  [unwired: 3 out]
    }
  }
  "Matches (Geometric Matching 6)" <- w9
  n95 = call <vilib>:"IVA Store Match Geometric Pattern Results.vi"("Calibrated Matches"=w8, "error in (no error)"=w11, "Matches"=w9, "Step Name"=w4, "Image in"=w6) -> ("error out"=w10:errorcluster, "Image dup"=→"Image Out":T5)  [unwired: 5 out]
  n96 = property on="Image Out" class="ImageControl"(error in=w10, "Palette:Palette Type"=w2) -> (error out=→"error out":errorcluster)  [unwired: 1 in, 1 out]
